vi "BotSpeak_System.vi"(2 "Values sent":i16[](array[numeric]), 3 "Variable In":string="power", 4 "Bot Settings":T1) -> (0 "response":string, 1 "Bot Settings":T1)   [LabVIEW 2012]
doc: "Writes the specified \"State\" (High or Low enumerated constant) to the specified \"DIO Line\""
uses:
  <userlib>/BotSpeak/VIs/Direct/BotSpeak_Control.ctl
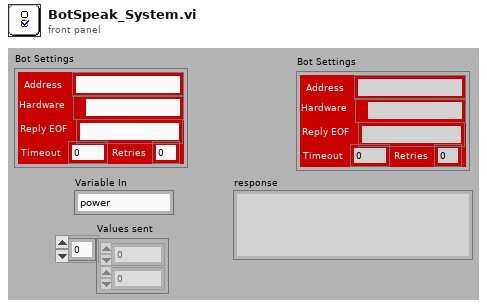
[diagram p1: front panel]
types:
  T1 = typedef "BotSpeak_Control.ctl" = cluster{"Address":string, "Reply EOF":string, "Hardware":path, "Retries":i8, "Timeout":i32}
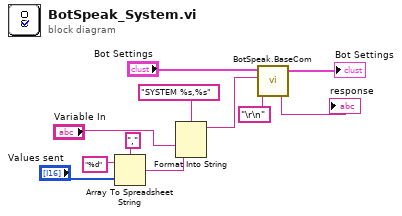
[diagram p0: block diagram]
diagram:
  n1 = Array To Spreadsheet String(delimiter (Tab)=",", array="Values sent", 3:"%d" ("format string")) -> (spreadsheet string=w3:string)
  n2 = Format Into String(format string="SYSTEM %s,%s" ("command"), "Variable In", w3) -> (resulting string=w11:string)  [unwired: 2 in, 1 out]
  n3 = call <userlib>:"BotSpeak.BaseCom.vi"("Termination"="\r\n", "command"=w11, "Bot Settings in"="Bot Settings") -> ("response"=→"response":string, "Bot Settings out"=→"Bot Settings":T1)  [unwired: 2 in]
